vi "sbRIO-9651.DAC Example.FPGA Main.vi"() -> ()   [LabVIEW 2015]
doc: "This is the main FPGA VI for the SPI application. It sets up the SPI communication and then runs the SPI engine. In a parallel loop, data is continually read from the Real Time application and sent to the SPI engine. The SPI engine handles all communication between the FPGA and the SPI chip."
uses:
  <vilib>/Platform/TimedLoop/XDataNode/timing_clust.ctl
  <vilib>/Platform/TimedLoop/XDataNode/nitl_modes.ctl
  <vilib>/Platform/TimedLoop/XDataNode/wakeup.ctl
  <vilib>/SPI API/vi.lib/SPI API/Controls/SPI Digital IO Lines.ctl
  <vilib>/SPI API/vi.lib/SPI API/Controls/SPI Digital IO Enable Lines.ctl
  <vilib>/rvi/Emulation/niFpgaGetClockAttributes.vi
  <vilib>/rvi/Emulation/niFpgaSctlEmulationGetInTimedLoop.vi
  <vilib>/rvi/Emulation/niFpgaEmulationReportErrorSimple.vi
  <vilib>/SPI API/vi.lib/SPI API/Polymorphic VI Instances/Initialize SPI Engine Resources 64-bit.vi
  <vilib>/rvi/Emulation/niFpgaCriticalErrorInLSC.vi
  <vilib>/SPI API/vi.lib/SPI API/Polymorphic VI Instances/SPI Engine 64-bit.vi
  <vilib>/SPI API/vi.lib/SPI API/Polymorphic VI Instances/Is SPI Engine Ready for Next Transaction 64-bit.vi
  <vilib>/SPI API/vi.lib/SPI API/Polymorphic VI Instances/Set SPI Transfer Length 64-bit.vi
  <vilib>/SPI API/vi.lib/SPI API/Polymorphic VI Instances/Set SPI Engine SCLK Divisor 64-bit.vi
  <vilib>/SPI API/vi.lib/SPI API/Polymorphic VI Instances/Set Data to Write for SPI Transaction 64-bit.vi
  <vilib>/SPI API/vi.lib/SPI API/Polymorphic VI Instances/Set Chip Select 64-bit.vi
  <vilib>/SPI API/vi.lib/SPI API/Polymorphic VI Instances/Start SPI Transaction 64-bit.vi
  <vilib>/SPI API/vi.lib/SPI API/Polymorphic VI Instances/Read SPI Response for SPI Transactions 64-bit.vi
  <vilib>/Platform/TimedLoop/XDataNode/XDataNode.xnode
  <vilib>/Platform/TimedLoop/XDataNode/XDNodeRunTimeDep.lvlib
  <vilib>/SPI API/vi.lib/SPI API/SPI API.lvlib
panel:
  in  "SPI Engine Clock Divisor":u8=42
  in  "Transfer Length (bits)":u8=32
  out "MOSI":bool
  out "SCLK":bool
  out "CS":bool
  out "Slave Response":u64
  out "read Iterations":i32
  in  "Data To Write":u64=2147483648
  in  "Chip Select":u8
  in  "Sample Rate (S/s)":u32=10000
  out "oclk freq":u32
  out "oclk div":u32
  out "Actual Loop Ticks":u32
  # "Overview: This is the FPGA VI that communicates with the MAX5216.\nRequirements: LabVIEW Full Development System, LabVIEW Real Time,  LabVIEW FPGA, MAX5216, NI System on Module, NI 9651.\nInstructions:\nRun RT Main without making adjustments to this VI to avoid a recompile.  If you desire to adjust this VI, do so, \nthen be sure to point RT Main to this VI instead of the pre-compiled bitfile that it currently targets."
  # "OUTPUT"
  # "INPUT"
  # "ADC Data::Debug"
  # "Acquisition Parameters"
  # "SPI Settings"
  # "Debug"
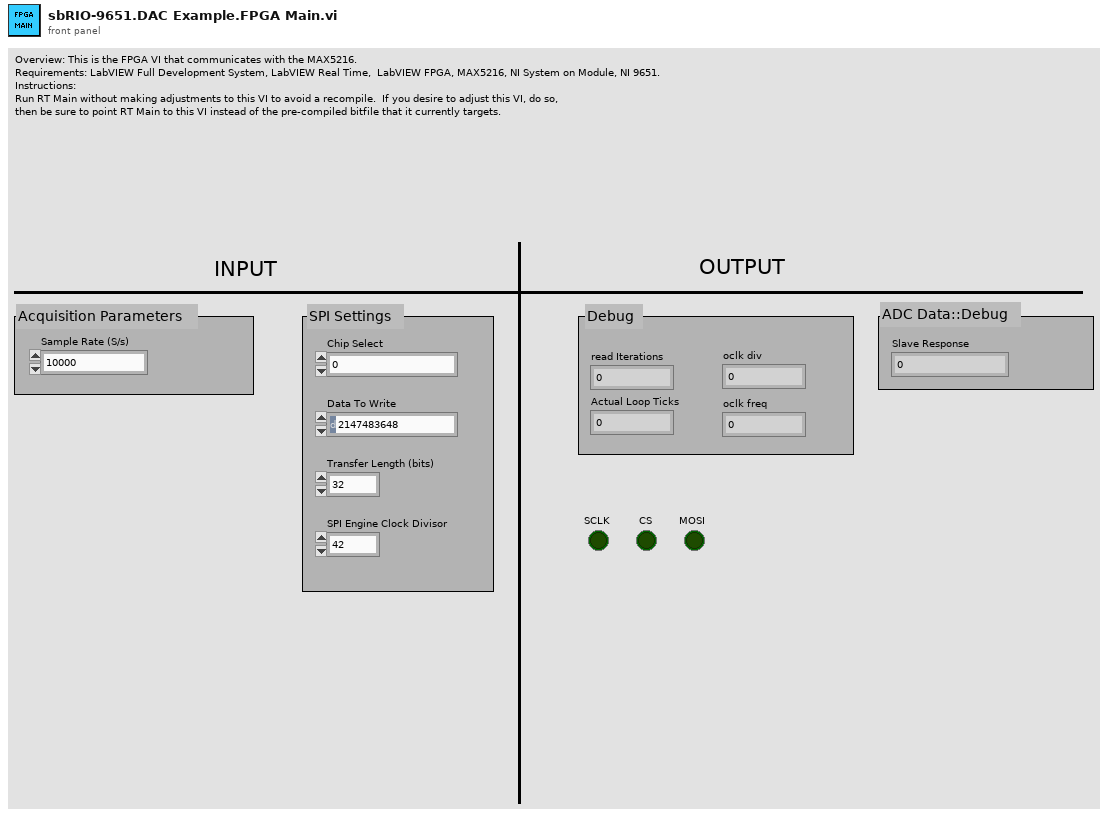
[diagram p1: front panel]
types:
  T1 = typedef "SPI API.lvlib/SPI Digital IO Enable Lines.ctl" = cluster{"SCLK_en":refnum<k21>, "MISO_en":refnum<k21>, "MOSI_en":refnum<k21>, "CS0_en":refnum<k21>, "CS1_en":refnum<k21>, "CS2_en":refnum<k21>, "CS3_en":refnum<k21>, "CS4_en":refnum<k21>, "CS5_en":refnum<k21>}
  T2 = typedef "SPI API.lvlib/SPI Digital IO Lines.ctl" = cluster{"SCLK":refnum<k21>, "MISO":refnum<k21>, "MOSI":refnum<k21>, "CS 0":refnum<k21>, "CS 1":refnum<k21>, "CS 2":refnum<k21>, "CS 3":refnum<k21>, "CS 4":refnum<k21>, "CS 5":refnum<k21>}
  T3 = typedef "SPI API.lvlib/SPI Engine Resources 64-bit.ctl" = cluster{"To SPI Engine Data FIFO":refnum<k21>, "From SPI Engine Data FIFO":refnum<k21>, "Data to SPI Engine Cache Register":refnum<k21>, "SPI Transaction Settings Cache Register":refnum<k21>}
  T4 = typedef "XDNodeRunTimeDep.lvlib/timing_clust.ctl" = cluster{"Expected End [f-1]":u64, "Actual End [f-1]":u64, "Finished Late? [f-1]":bool, "Expected End [i-1]":u64, "Actual End [i-1]":u64, "Finished Late? [i-1]":bool, "Expected Start [i]":u64, "Actual Start [i]":u64, "Expected Start [f]":u64, "Actual Start [f]":u64, "Source Name":string, "Structure Name":string, "Period":i64, "Deadline":i64, "Offset":i64, "Start":i64, "Priority":i32, "Timeout":i32, "Mode":T5, "Wakeup Reason":T6, "Error":errorcluster, "Source Type":string, "Secondary Source Type":string, "Global End Time":u64, "Global Start Time":u64, "Frame Duration":u64, "Iteration Duration":u64, "Assigned CPU":i32, "I/O Scan Engine Mode":u32}
  T5 = typedef "XDNodeRunTimeDep.lvlib/nitl_modes.ctl" = enum32{"No Change", "Process missed periods, maintain original phase", "Discard missed periods, maintain original phase", "Process missed periods, ignore original phase", "Discard missed periods, ignore original phase"}
  T6 = typedef "XDNodeRunTimeDep.lvlib/wakeup.ctl" = enum32{"Normal", "Aborted", "Asynchronous wakeup", "Timing source error", "Timed loop error", "Timeout"}
  T7 = typedef "SPI API.lvlib/SPI API Response Data 64-bit.ctl" = cluster{"Response Data":T8, "Node Id":u16}
  T8 = typedef "SPI API.lvlib/SPI API Data 64-bit.ctl" = bool[]
  T9 = typedef "NI SPI IP FPGA.lvlib/Spi Master Inputs.ctl" = cluster{"MISO":bool}
  T10 = typedef "NI SPI IP FPGA.lvlib/Spi Master Outputs.ctl" = cluster{"Chip Select":bool, "Clock":bool, "MOSI":bool, "MOSI OE":bool}
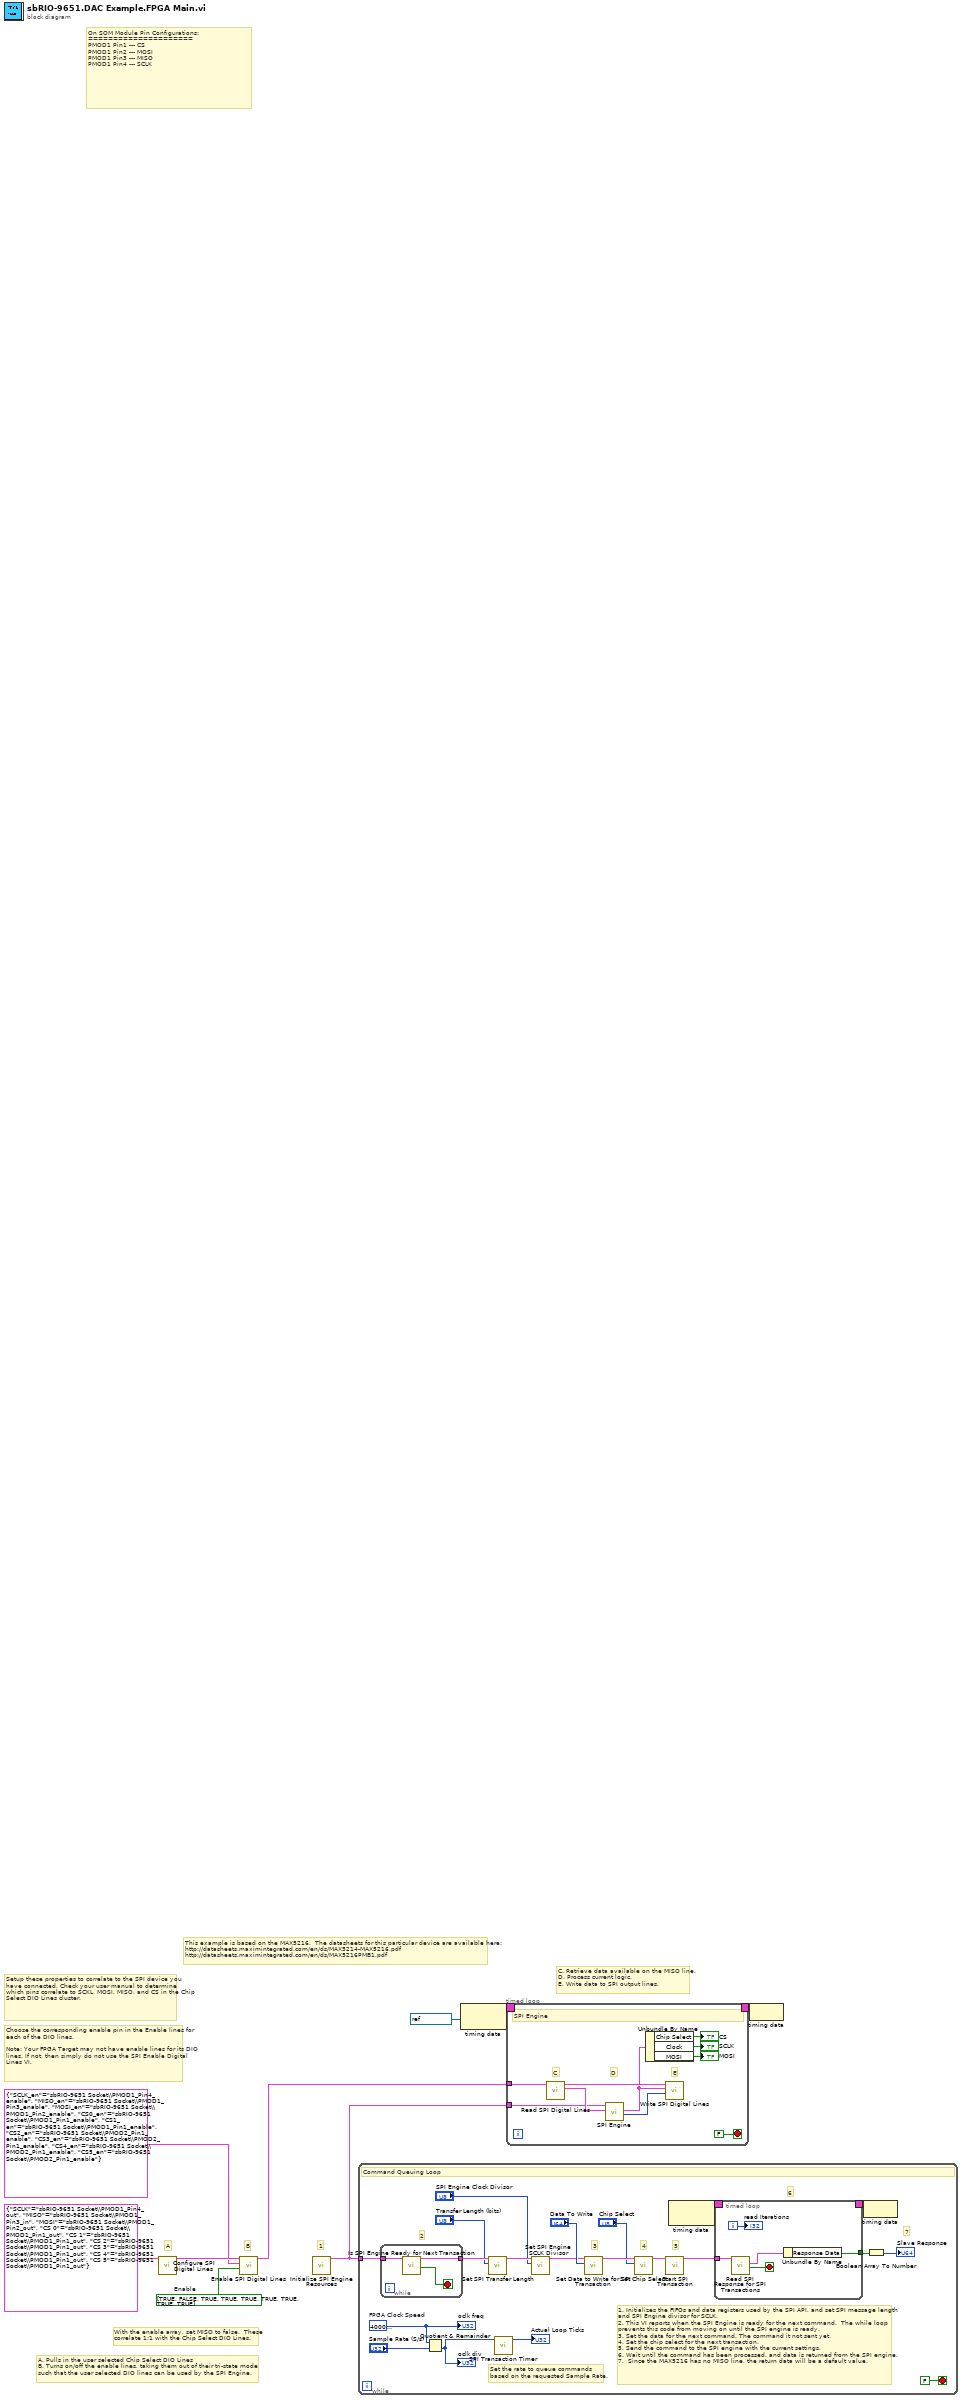
[diagram p0: block diagram]
diagram:
  w2 = bool[] [TRUE, FALSE, TRUE, TRUE, TRUE, TRUE, TRUE, TRUE, TRUE]  # Enable
  # "Choose the corresponding enable pin in the Enable lines for each of the DIO lines.\n\nNote: Your FPGA Target may not have enable lines for its DIO lines. If not, then simply do not use the SPI Enable Digital Lines VI."
  # "With the enable array, set MISO to false.  These\ncorrelate 1:1 with the Chip Select DIO Lines."
  # "A. Pulls in the user selected Chip Select DIO Lines\nB. Turns on/off the enable lines, taking them out of their tri-state mode \nsuch that the user selected DIO lines can be used by the SPI Engine."
  # "This example is based on the MAX5216.  The datasheets for this particular device are available here:\nhttp://datasheets.maximintegrated.com/en/ds/MAX5214-MAX5216.pdf\nhttp://datasheets.maximintegrated.com/en/ds/MAX5216PMB1.pdf"
  # "C. Retrieve data available on the MISO line.\nD. Process current logic.\nE. Write data to SPI output lines."
  # "B"
  # "A"
  # "1"
  # "Setup these properties to correlate to the SPI device you have connected. Check your user manual to determine which pins correlate to SCKL, MOSI, MISO, and CS in the Chip Select DIO Lines cluster."
  # "On SOM Module Pin Configurations:\n=====================\nPMOD1 Pin1 --- CS\nPMOD1 Pin2 --- MOSI\nPMOD1 Pin3 --- MISO\nPMOD1 Pin4 --- SCLK"
  n1 = call <vilib>:"Configure SPI Digital Lines.vi"("SPI Digital I/O Lines"=T2 {"SCLK"="sbRIO-9651 Socket\\PMOD1_Pin4_out", "MISO"="sbRIO-9651 Socket\\PMOD1_Pin3_in", "MOSI"="sbRIO-9651 Socket\\PMOD1_Pin2_out", "CS 0"="sbRIO-9651 Socket\\PMOD1_Pin1_out", "CS 1"="sbRIO-9651 Socket\\PMOD1_Pin1_out", "CS 2"="sbRIO-9651 Socket\\PMOD1_Pin1_out", "CS 3"="sbRIO-9651 Socket\\PMOD1_Pin1_out", "CS 4"="sbRIO-9651 Socket\\PMOD1_Pin1_out", "CS 5"="sbRIO-9651 Socket\\PMOD1_Pin1_out"}) -> ("SPI Digital I/O Lines"=w5:T2)  [unwired: 9 in, 1 out]
  n2 = call <vilib>:"Enable SPI Digital Lines.vi"("Enable Lines States"=w2, "Enable Lines"=T1 {"SCLK_en"="sbRIO-9651 Socket\\PMOD1_Pin4_enable", "MISO_en"="sbRIO-9651 Socket\\PMOD1_Pin3_enable", "MOSI_en"="sbRIO-9651 Socket\\PMOD1_Pin2_enable", "CS0_en"="sbRIO-9651 Socket\\PMOD1_Pin1_enable", "CS1_en"="sbRIO-9651 Socket\\PMOD1_Pin1_enable", "CS2_en"="sbRIO-9651 Socket\\PMOD2_Pin1_enable", "CS3_en"="sbRIO-9651 Socket\\PMOD2_Pin1_enable", "CS4_en"="sbRIO-9651 Socket\\PMOD2_Pin1_enable", "CS5_en"="sbRIO-9651 Socket\\PMOD2_Pin1_enable"}, "SPI Digital I/O Lines"=w5) -> ("SPI Digital I/O Lines"=w3:T2)  [unwired: 7 in, 1 out]
  n3 = call-poly <vilib>:"Initialize SPI Engine Resources.vi"() -> ("SPI Engine Resources 64-bit"=w1:T3)  [unwired: 10 in, 1 out]
  n4 = while {
    tunnel: w1 -> [w16]
    stop <- FALSE stop-if-true
    w26 = u32 40000000  # FPGA Clock Speed
    # "1. Initializes the FIFOs and data registers used by the SPI API, and set SPI message length\nand SPI Engine divisor for SCLK.\n2. This VI reports when the SPI Engine is ready for the next command.  The while loop \nprevents this code from moving on until the SPI engine is ready.\n3. Set the data for the next command. The command it not sent yet.\n4. Set the chip select for the next transaction.\n5. Send the command to the SPI engine with the current settings.\n6. Wait until the command has been processed, and data is returned from the SPI engine.\n7.  Since the MAX5216 has no MISO line, the return data will be a default value."
    # "Set the rate to queue commands\nbased on the requested Sample Rate."
    # "7"
    # "6"
    # "5"
    # "4"
    # "3"
    # "2"
    # "Command Queuing Loop"
    n5 = while {
      tunnel: [w32] -> w14
      tunnel: w16 -> [w30]
      stop <- w31 stop-if-true
      n6 = call-poly <vilib>:"Is SPI Engine Ready for Next Transaction.vi"("SPI Engine Resources"=w30) -> ("SPI Engine Ready?"=w31:bool, "SPI Engine Resources"=w32:T3)  [unwired: 7 in, 2 out]
    }
    n7 = Quotient & Remainder(x=w26, y="Sample Rate (S/s)") -> (floor(x/y)=w15:u32)  [unwired: 1 out]
    "oclk div" <- w15
    n8 = call-poly <vilib>:"Set SPI Transfer Length.vi"("Transfer Length (bits)"="Transfer Length (bits)", "SPI Engine Resources"=w14) -> ("SPI Engine Resources"=w13:T3)  [unwired: 8 in, 1 out]
    n9 = call <vilib>:"SPI Transaction Timer.vi"("Loop Time (Ticks)"=w15) -> ("Actual Time (Ticks)"=→"Actual Loop Ticks":u32)  [unwired: 10 in]
    n10 = call-poly <vilib>:"Set SPI Engine SCLK Divisor.vi"("SPI Engine Clock Divisor"="SPI Engine Clock Divisor", "SPI Engine Resources"=w13) -> ("SPI Engine Resources"=w12:T3)  [unwired: 7 in, 2 out]
    n11 = call-poly <vilib>:"Set Data to Write for SPI Transaction.vi"("Data In"="Data To Write", "SPI Engine Resources"=w12) -> ("SPI Engine Resources"=w20:T3)  [unwired: 8 in, 1 out]
    n12 = call-poly <vilib>:"Set Chip Select.vi"("Chip Select"="Chip Select", "SPI Engine Resources"=w20) -> ("SPI Engine Resources"=w19:T3)  [unwired: 8 in, 1 out]
    n13 = call-poly <vilib>:"Start SPI Transaction.vi"("SPI Engine Resources"=w19) -> ("SPI Engine Resources"=w24:T3)  [unwired: 8 in, 2 out]
    n14 = node-c288() -> (w29:T4)  [unwired: 1 in]
    n15 = timed-loop {
      timing: w29 -> [_]
      timing-out: [_] -> w28
      tunnel: w24 -> [w33]
      tunnel: [w36] -> w22
      i -> [w37]
      stop <- w34 stop-if-true
      n16 = call-poly <vilib>:"Read SPI Response for SPI Transactions.vi"("SPI Engine Resources"=w33) -> ("Read Data Valid?"=w34:bool, "Read Data"=w35:T7)  [unwired: 7 in, 2 out]
      n17 = Unbundle By Name(w35) -> ("Response Data"=w36:T8)
      "read Iterations" <- w37
    }
    n18 = node-c288(w28) -> ()
    n19 = Boolean Array To Number(Boolean array=w22) -> (number=→"Slave Response":u64)
    "oclk freq" <- w26
  }
  n20 = node-c288(refnum<k21> "120MHz" ("Source Name")) -> (w9:T4)
  n21 = timed-loop {
    tunnel: w1 -> [w46]
    tunnel: w3 -> [w50]
    timing: w9 -> [_]
    timing-out: [_] -> w8
    stop <- FALSE stop-if-true
    # "E"
    # "D"
    # "C"
    # "SPI Engine"
    n22 = call <vilib>:"Read SPI Digital Lines.vi"("SPI Digital I/O Lines"=w50) -> ("SPI Read Data"=w48:T9, "SPI Digital I/O Lines"=w49:T2)  [unwired: 8 in, 1 out]
    n23 = call-poly <vilib>:"SPI Engine.vi"("SPI Read Data"=w48, "SPI Engine Resources"=w46) -> ("Chip Select"=w47:u8, "SPI Write Data"=w45:T10)  [unwired: 6 in, 2 out]
    n24 = Unbundle By Name(w45) -> ("Chip Select"=→"CS":bool, "Clock"=→"SCLK":bool, "MOSI"=→"MOSI":bool)
    n25 = call <vilib>:"Write SPI Digital Lines.vi"("Chip Select"=w47, "SPI Write Data"=w45, "SPI Digital I/O Lines"=w49) -> ()  [unwired: 7 in, 2 out]
  }
  n26 = node-c288(w8) -> ()
